vi "Tektronix AFG 3000 Series Frequency Sweep.vi"() -> ()   [LabVIEW 2009, in "Tektronix AFG 3000 Series.lvlib"]
doc: "Demonstrates how to configure and enable a frequency sweep."
uses:
  Tektronix AFG 3000 Series.lvlib
panel:
  in  "Channel (0: Channel 1)":u16(ring) items=["Channel 1", "Channel 2"]
  in  "Amplitude (1 Vpp)":dbl[unit]=1.0
  in  "Waveform Function (0: Sine)":u16(ring) items=["Sine", "Square", "Pulse", "Ramp", "Noise", "DC", "Sin(x)/x", "Gaussian", "Lorentz", "Exponential Rise", "Exponential Decay", "Haversine"]
  in  "Stop  Frequency  (1000 Hz)":dbl[unit]=1000.0 format="%#.6g"
  in  "Start Frequency (100 Hz)":dbl[unit]=100.0 format="%#.6g"
  in  "Sweep Time (1.00 s)":dbl[unit]=1.0 format="%#.6g"
  in  "VISA resource name":refnum<visa-resource-name>
  # "(c) 2006-2009 National Instruments.  ALL RIGHTS RESERVED."
  # "The Pulse, Noise, and DC waveform functions are not valid for Frequency Sweep."
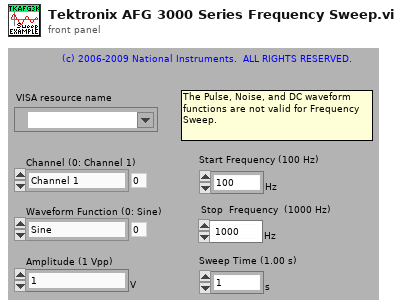
[diagram p1: front panel]
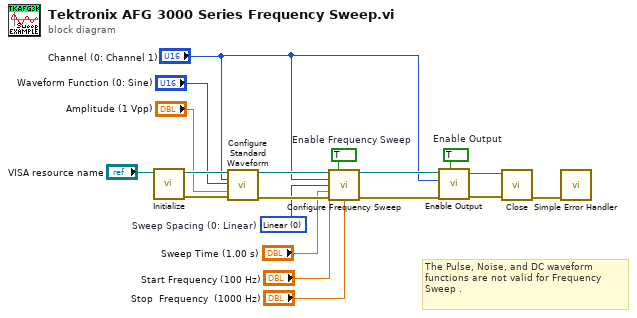
[diagram p0: block diagram]
diagram:
  w4 = TRUE  # Enable Output
  w5 = u16 0 items=["Linear", "Log"]  # Sweep Spacing (0: Linear)
  w11 = TRUE  # Enable Frequency Sweep
  # "The Pulse, Noise, and DC waveform functions are not valid for Frequency Sweep ."
  n1 = call "Initialize.vi"("VISA resource name"="VISA resource name") -> ("error out"=w15:errorcluster, "VISA resource name out"=w19:refnum<visa-resource-name>)  [unwired: 4 in, 5 out]
  n2 = call "Configure Standard Waveform.vi"("VISA resource name"=w19, "Channel (0: Channel 1)"="Channel (0: Channel 1)", "Waveform Function (0: Sine)"="Waveform Function (0: Sine)", "Amplitude (1 Vpp)"="Amplitude (1 Vpp)", "error in (no error)"=w15) -> ("VISA resource name out"=w16:refnum<visa-resource-name>, "error out"=w17:errorcluster)  [unwired: 2 in, 7 out]
  n3 = call "Configure Frequency Sweep.vi"("VISA resource name"=w16, "Enable Frequency Sweep (T: Enable)"=w11, "Channel (0: Channel 1)"="Channel (0: Channel 1)", "Sweep Spacing (0: Linear)"=w5, "Sweep Time (1.00 s)"="Sweep Time (1.00 s)", "error in (no error)"=w17, "Start Frequency (100 Hz)"="Start Frequency (100 Hz)", "Stop  Frequency  (1000 Hz)"="Stop  Frequency  (1000 Hz)") -> ("VISA resource name out"=w3:refnum<visa-resource-name>, "error out"=w2:errorcluster)  [unwired: 6 out]
  n4 = call "Enable Output.vi"("Enable Output (T: Enable)"=w4, "error in (no error)"=w2, "Channel (0: Channel 1)"="Channel (0: Channel 1)", "VISA resource name"=w3) -> ("error out"=w14:errorcluster, "VISA resource name out"=w13:refnum<visa-resource-name>)  [unwired: 6 out]
  n5 = call "Close.vi"("error in (no error)"=w14, "VISA resource name"=w13) -> ("error out"=w18:errorcluster)  [unwired: 9 out]
  n6 = call <vilib>:"Simple Error Handler.vi"("error in (no error)"=w18) -> ()  [unwired: 1 in, 8 out]
